vi "dataset.create_add_label.vi"(8 "error in":errorcluster, 11 "DatasetCreateStaging in":refnum<class "DatasetCreateStaging.lvclass">) -> (0 "error out":errorcluster, 3 "DatasetCreateStaging out":refnum<class "DatasetCreateStaging.lvclass">)   [LabVIEW 2020, in "DatasetCreateStaging.lvclass"]
doc: "Adds a label to the dataset being created."
uses:
  DatasetCreateStaging.lvclass
  DatasetCreateStaging.lvclass/DatasetCreateStaging.ctl
  client.lvlib
panel:
  in  "label":string
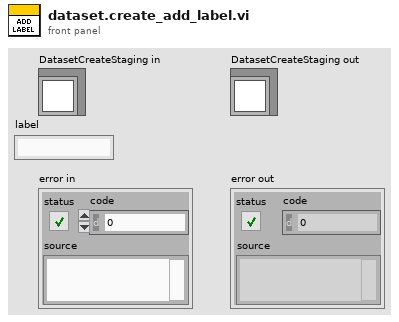
[diagram p1: front panel]
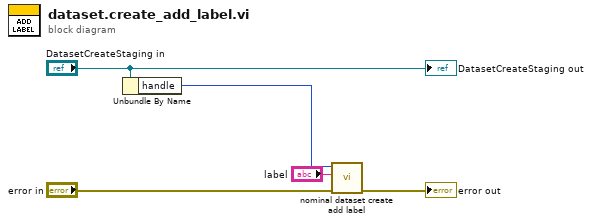
[diagram p0: block diagram]
diagram:
  n1 = Unbundle By Name("DatasetCreateStaging in") -> ("handle"=w3:i32)
  n2 = call "nominal dataset create add label.vi"("error in (no error)"="error in", "label"="label", "staging"=w3) -> ("error out"=→"error out":errorcluster)  [unwired: 7 in, 1 out]
  "DatasetCreateStaging out" <- "DatasetCreateStaging in"
